vi "Test.vi"() -> ()   [LabVIEW 2009]
panel:
  out "Result":string
  out "Value":string
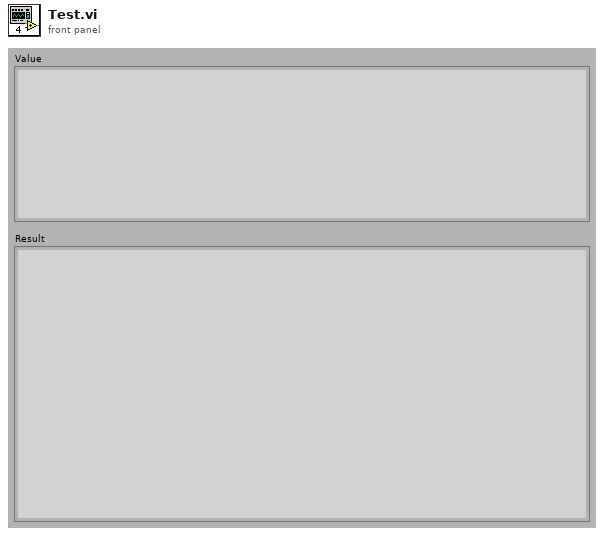
[diagram p1: front panel]
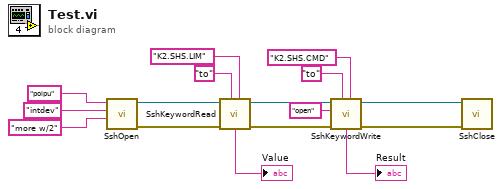
[diagram p0: block diagram]
diagram:
  n1 = call "SshOpen.vi"("host"="poipu", "username"="intdev", "password"="more w/2") -> ("SshStream"=w13:refnum<k24>, "error out"=w12:errorcluster)  [unwired: 2 in, 3 out]
  n2 = call "SshKeywordRead.vi"("error in (no error)"=w12, "SshStream in"=w13, "Service"="to" ("entrée1"), "Keyword"="K2.SHS.LIM" ("entrée2")) -> ("Result"=→"Value":string, "error out"=w8:errorcluster, "SshStream out"=w4:refnum<k24>)  [unwired: 2 in, 2 out]
  n3 = call "SshKeywordWrite.vi"("error in (no error)"=w8, "Value"="open", "SshStream in"=w4, "Service"="to", "Keyword"="K2.SHS.CMD") -> ("Result"=→"Result":string, "error out"=w7:errorcluster, "SshStream out"=w3:refnum<k24>)  [unwired: 1 in, 2 out]
  n4 = call "SshClose.vi"("SshStream in"=w3, "error in (no error)"=w7) -> ()  [unwired: 8 out]
